vi "LSX Create LSID.vi"(8 "error in (no error)":errorcluster, 11 "plLSID":i32) -> (0 "error out":errorcluster, 2 "function return":i32, 3 "plLSID out":i32)   [LabVIEW 2016, in "Tango_DLL.lvlib"]
doc: "TANGOAPI int TANGOCALL LSX_CreateLSID (int *plLSID);"
uses:
  Tango_DLL.lvlib
  Tango_DLL.dll
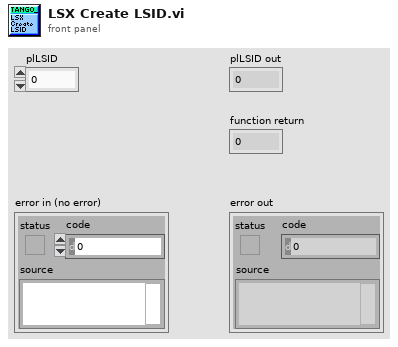
[diagram p1: front panel]
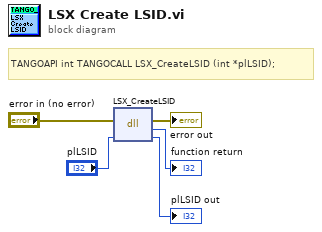
[diagram p0: block diagram]
diagram:
  # "TANGOAPI int TANGOCALL LSX_CreateLSID (int *plLSID);"
  n1 = dll-call lib="C:/Users/4PiSMS/Documents/Microscope Control/2016/Device Library/Stages/Marzhauser/SCAN IM 120 x 80/Tango DLL VIs/Tango_DLL.*" fn="LSX_CreateLSID"(error in="error in (no error)", "plLSID"="plLSID") -> (error out=→"error out":errorcluster, →"function return":i32, "plLSID"=→"plLSID out":i32)  [unwired: 2 in, 1 out]
